vi "GetHeightDistanceSensor.vi"(0 "controller in":refnum<k24>, 1 "error in (no error)":errorcluster) -> (2 "controller out":refnum<k24>, 3 "MeanHeight(mm)":dbl format="%0.3f", 4 "SDofHeight(mm)":dbl format="%0.3f", 5 "error out":errorcluster)   [LabVIEW 2021]
uses:
  C:/Users/TTUHEP/Documents/LabVIEW/Other Models/2010/Bin/Aerotech.A3200.dll
  Other Models/2010/Bin/Aerotech.A3200.dll
  <vilib>/Analysis/NI_AALBase.lvlib
panel:
  out "UnlockResult":string
  in  "Gcodes":string[](array[string])=["G1 X-0.25 Y-0.25 F1", "G1 X0.6 F1", "G1 Y0.4 F1", "G1 X-0.4 Y0.25 F1", "G1 X0.05 Y-0.4 F1"]
  out "Distances(mm)":dbl[](array[numeric])
  out "LockResult":string
  out "String":string
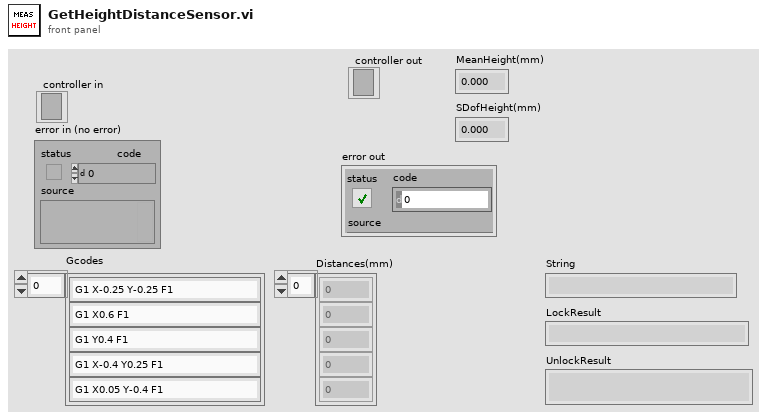
[diagram p1: front panel]
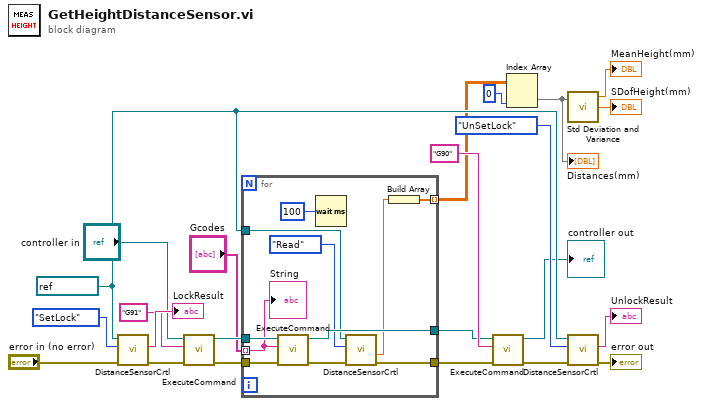
[diagram p0: block diagram]
diagram:
  w12 = refnum<visa-resource-name> "COM4" ("VISA resource name")
  n1 = call "DistanceSensorCrtl.vi"("error in (no error)"="error in (no error)", "Control Option"=enum16{"SetLock", "UnSetLock", "Read"}."SetLock", "VISA resource name"=w12) -> ("error out"=w20:errorcluster, "Result"=→"LockResult":string)  [unwired: 5 in, 2 out]
  n2 = call "ExecuteCommand.vi"("error in (no error)"=w20, "Command Code"="G91", "controller in"="controller in") -> ("error out"=w19:errorcluster, "controller out"=w18:refnum<k24>)  [unwired: 6 in, 1 out]
  n3 = for {
    tunnel: "Gcodes" -> [w30] mode=indexing
    tunnel: w19 -> [w33]
    tunnel: w18 -> [w32]
    tunnel: [w26] -> w15
    tunnel: [w31] -> w16
    tunnel: w12 -> [w27]
    tunnel: [w24] -> w9 mode=indexing
    n4 = call "ExecuteCommand.vi"("error in (no error)"=w33, "Command Code"=w30, "controller in"=w32) -> ("error out"=w29:errorcluster, "controller out"=w31:refnum<k24>)  [unwired: 6 in, 1 out]
    n5 = Wait (ms)(milliseconds to wait=u32 100) -> ()  [unwired: 1 out]
    n6 = call "DistanceSensorCrtl.vi"("error in (no error)"=w29, "Control Option"=enum16{"SetLock", "UnSetLock", "Read"}."Read", "VISA resource name"=w27) -> ("error out"=w26:errorcluster, "Distance(mm)"=w25:dbl)  [unwired: 5 in, 2 out]
    n7 = Build Array(w25) -> (w24:dbl[])
    "String" <- w30
  }
  n8 = call "ExecuteCommand.vi"("error in (no error)"=w15, "Command Code"="G90", "controller in"=w16) -> ("error out"=w13:errorcluster, "controller out"=→"controller out":refnum<k24>)  [unwired: 6 in, 1 out]
  n9 = Index Array(array=w9, index (col)=0 ("disabled index (col)")) -> (element=w5:dbl[])  [unwired: 1 in]
  "Distances(mm)" <- w5
  n10 = call <vilib>:"Std Deviation and Variance.vi"("X"=w5) -> ("mean"=→"MeanHeight(mm)":dbl, "standard deviation"=→"SDofHeight(mm)":dbl)  [unwired: 1 in, 1 out]
  n11 = call "DistanceSensorCrtl.vi"("error in (no error)"=w13, "Control Option"=enum16{"SetLock", "UnSetLock", "Read"}."UnSetLock", "VISA resource name"=w12) -> ("error out"=→"error out":errorcluster, "Result"=→"UnlockResult":string)  [unwired: 5 in, 2 out]
